vi "Image_to_Vector.vi"(0 "Image Pixels (U8)":u8[][](array[numeric]), 1 "Skip-1":i32=1) -> (2 "Final Index":i32, 3 "Y Size":i32, 4 "X Size":i32, 5 "Vector Format":i32[][](array[numeric]))   [LabVIEW 2009]
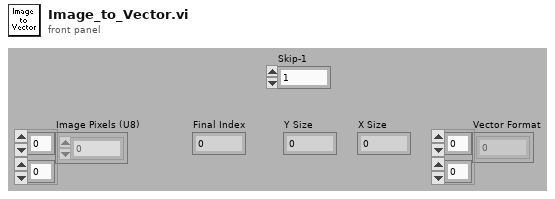
[diagram p1: front panel]
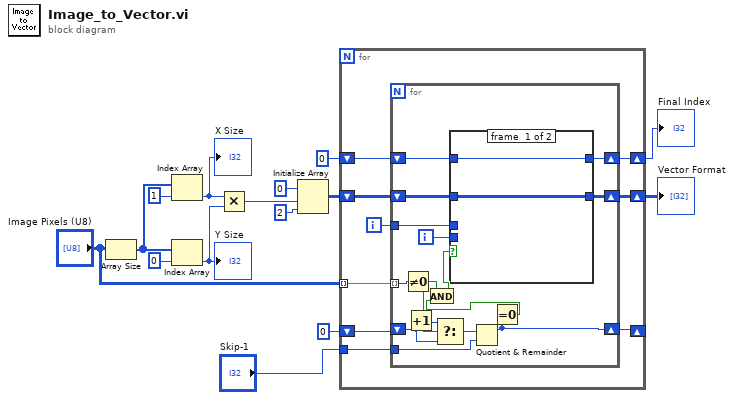
[diagram p0: block diagram]
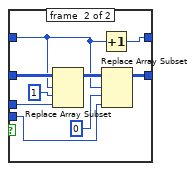
[diagram p2: hidden frame]
diagram:
  n1 = Array Size(array="Image Pixels (U8)") -> (size(s)=w3:i32[])
  n2 = Index Array(array=w3, index=1) -> (element=w15:i32)
  "X Size" <- w15
  n3 = Index Array(array=w3, index=0) -> (element=w14:i32)
  "Y Size" <- w14
  n4 = Multiply(x=w15, y=w14) -> (x*y=w13:i32)
  n5 = Initialize Array(0 ("element"), w13, 2 ("dimension size")) -> (w9:i32[][])
  n6 = for {
    tunnel: "Image Pixels (U8)" -> [w24] mode=indexing
    shift-right: [w22] -> w10
    shift-left: w9 -> [w23]
    shift-right: [w19] -> w12
    shift-left: 0 ("dimension size") -> [w20]
    shift-right: [w17] -> _
    shift-left: 0 ("dimension size") -> [w18]
    tunnel: "Skip-1" -> [w16]
    i -> [w21]
    n7 = for {
      tunnel: w24 -> [w33] mode=indexing
      shift-right: [w38] -> w22
      shift-left: w23 -> [w39]
      tunnel: w21 -> [w37]
      shift-right: [w34] -> w19
      shift-left: w20 -> [w35]
      shift-right: [w27] -> w17
      shift-left: w18 -> [w29]
      tunnel: w16 -> [w26]
      i -> [w36]
      n8 = Not Equal To 0?(x=w33) -> (x != 0?=w32:bool)
      n9 = Increment(x=w29) -> (x+1=w30:i32)
      n10 = Select(t=w30, s=w32, f=w29) -> (s? t:f=w28:i32)
      n11 = Quotient & Remainder(x=w28, y=w26) -> (x-y*floor(x/y)=w27:i32)  [unwired: 1 out]
      n12 = Equal To 0?(x=w27) -> (x = 0?=w31:bool)
      n13 = And(x=w32, y=w31) -> (x .and. y?=w25:bool)
      n14 = case shown="True" w25 {
        tunnel: w39 -> [w41 w50]
        tunnel: [w41 w47] -> w38
        tunnel: w37 -> [_ w43]
        tunnel: w36 -> [_ w42]
        tunnel: w35 -> [w40 w45]
        tunnel: [w40 w49] -> w34
        frame #0 {
        }
        frame #1 {
          n15 = Replace Array Subset(array=w50, new element=w43, index (row)=w45, index (col)=1 ("disabled index (col)")) -> (w48:i32[][])
          n16 = Increment(x=w45) -> (x+1=w49:i32)
          n17 = Replace Array Subset(array=w48, new element=w42, index (row)=w45, index (col)=0 ("disabled index (col)")) -> (w47:i32[][])
        }
      }
    }
  }
  "Final Index" <- w12
  "Vector Format" <- w10
